vi "Write I64.vi"(8 "error in (no error)":errorcluster, 9 "Data":i64, 10 "Channel Name":string, 11 "CIFChannelMng in":refnum<class "CIFChannelMng.lvclass">) -> (0 "error out":errorcluster, 1 "timed out?":bool, 3 "CIFChannelMng out":refnum<class "CIFChannelMng.lvclass">)   [LabVIEW 2021, in "CIFChannelMng.lvclass"]
uses:
  CIFChannelMng.lvclass
  CIFChannelMng.lvclass/CIFChannelMng.ctl
  CIFClocks/Typedef/Errors.ctl
  <vilib>/Utility/miscctls.llb/LVMapReplaceAction.ctl
  CIFCore/Common/Utilities/Append Error Location.vi
  CIFChannels/CIFChannels.lvclass
  CIFCore/Common/CIFCoreCommon.lvlib
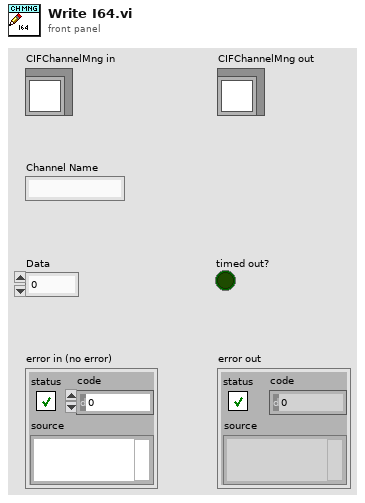
[diagram p1: front panel]
types:
  T1 = typedef "CIFCoreCommon.lvlib/Errors.ctl" = enum16{"Invalid Clock ID", "Long Sleep", "gRPC Server Not Found", "Config Parse", "Timestamp Wrap", "Delayed Execution", "Duplicate Channel", "Missing Channel", "Incorrect Type", "Unregistered Enum"}
  T2 = typedef "LVMapReplaceAction.ctl" = enum32{"Modify Entry only if found", "Add or Modify Entry", "Delete Entry"}
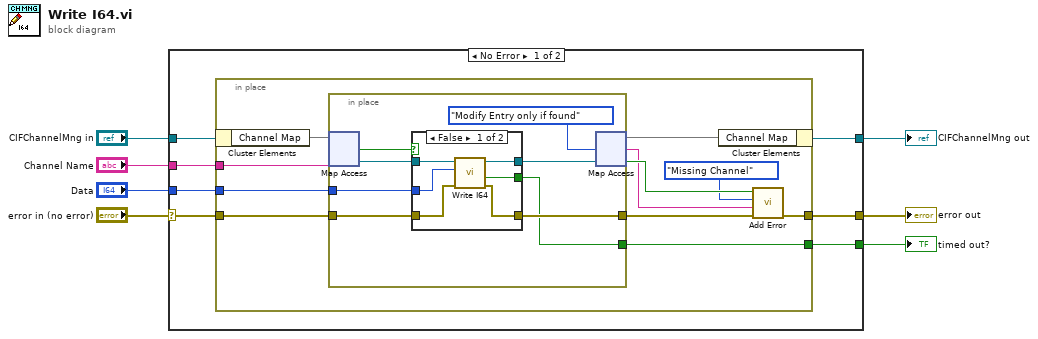
[diagram p0: block diagram]
diagram:
  n1 = case shown="No Error" "error in (no error)" {
    selector: "error in (no error)" -> [w12 w43]
    tunnel: [w10 w43] -> w6
    tunnel: [w13 w42] -> w4
    tunnel: "CIFChannelMng in" -> [w14 w42]
    tunnel: "Channel Name" -> [w11 _]
    tunnel: "Data" -> [w9 _]
    tunnel: [w8 _] -> w1
    frame No Error {
      n2 = in-place {
        in-place-border: w11 -> [w19]
        in-place-border: w12 -> [w23]
        in-place-border: [w20] -> w10
        in-place-border: w9 -> [w16]
        in-place-border: [w15] -> w8
        n3 = in-place-cluster #1(w14) -> ("Channel Map"=w25:map{string, refnum<class "CIFChannels.lvclass">})
        n4 = in-place {
          in-place-border: w23 -> [w30]
          in-place-border: [w29] -> w21
          in-place-border: [w27] -> w15
          in-place-border: w16 -> [w26]
          n5 = in-place-map #2(w25, w19) -> (w32:refnum<class "CIFChannels.lvclass">, w28:bool)  [unwired: 1 in]
          n6 = case shown="False" w28 {
            tunnel: w32 -> [w39 w41]
            tunnel: [w38 w41] -> w31
            tunnel: w30 -> [w37 w40]
            tunnel: [w36 w40] -> w29
            tunnel: [w35 _] -> w27
            tunnel: w26 -> [w34 _]
            frame False {
              n7 = call-dynamic "Write I64.vi"("error in (no error)"=w37, "Data"=w34, "CIFChannels in"=w39) -> ("error out"=w36:errorcluster, "timed out?"=w35:bool, "CIFChannels out"=w38:refnum<class "CIFChannels.lvclass">)  [unwired: 6 in]
            }
            frame True {
            }
          }
          n8 = in-place-map #2(w31, LVMapReplaceAction."Modify Entry only if found" ("action")) -> (w24:map{string, refnum<class "CIFChannels.lvclass">}, w18:string, w22:bool)
        }
        n9 = in-place-cluster #1("Channel Map"=w24) -> (w13:refnum<class "CIFChannelMng.lvclass">)
        n10 = call "Add Error.vi"("error in (no error)"=w21, "String to Append"=w18, "Error"=Errors."Missing Channel", "Insert Error"=w22) -> ("error out"=w20:errorcluster)  [unwired: 7 in]
      }
    }
    frame Error {
    }
  }
  "error out" <- w6
  "CIFChannelMng out" <- w4
  "timed out?" <- w1
